vi "test.vi"(8 "error in (no error)":errorcluster, 11 "DAQOrcaFlash in":refnum<class "DAQOrcaFlash.lvclass">) -> (0 "error out":errorcluster, 3 "DAQOrcaFlash out":refnum<class "DAQOrcaFlash.lvclass">)   [LabVIEW 2012, in "DAQOrcaFlash.lvclass"]
uses:
  DAQOrcaFlash.lvclass
  <vilib>/vision/NI_Vision_Development_Module.lvlib
panel:
  out "max value 4":sgl
  out "min value 4":sgl
  out "max value 3":sgl
  out "min value 3":sgl
  out "min value":sgl
  out "max value":sgl
  in  "Path":path
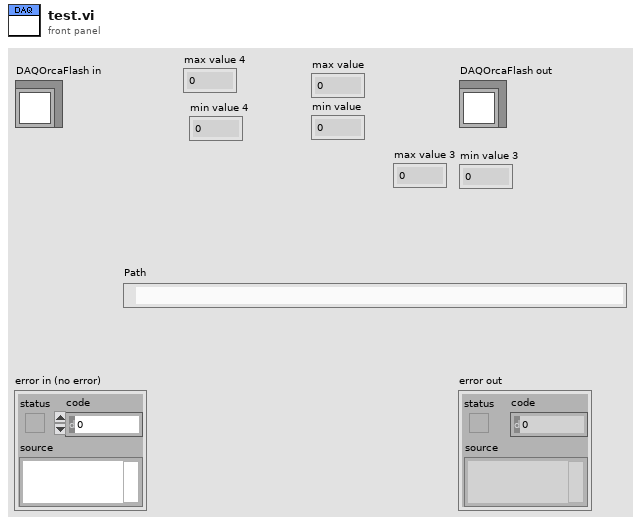
[diagram p1: front panel]
types:
  T1 = typedef "Image Type" = u32
  T2 = typedef "IMAQ Image.ctl" = refnum<image>
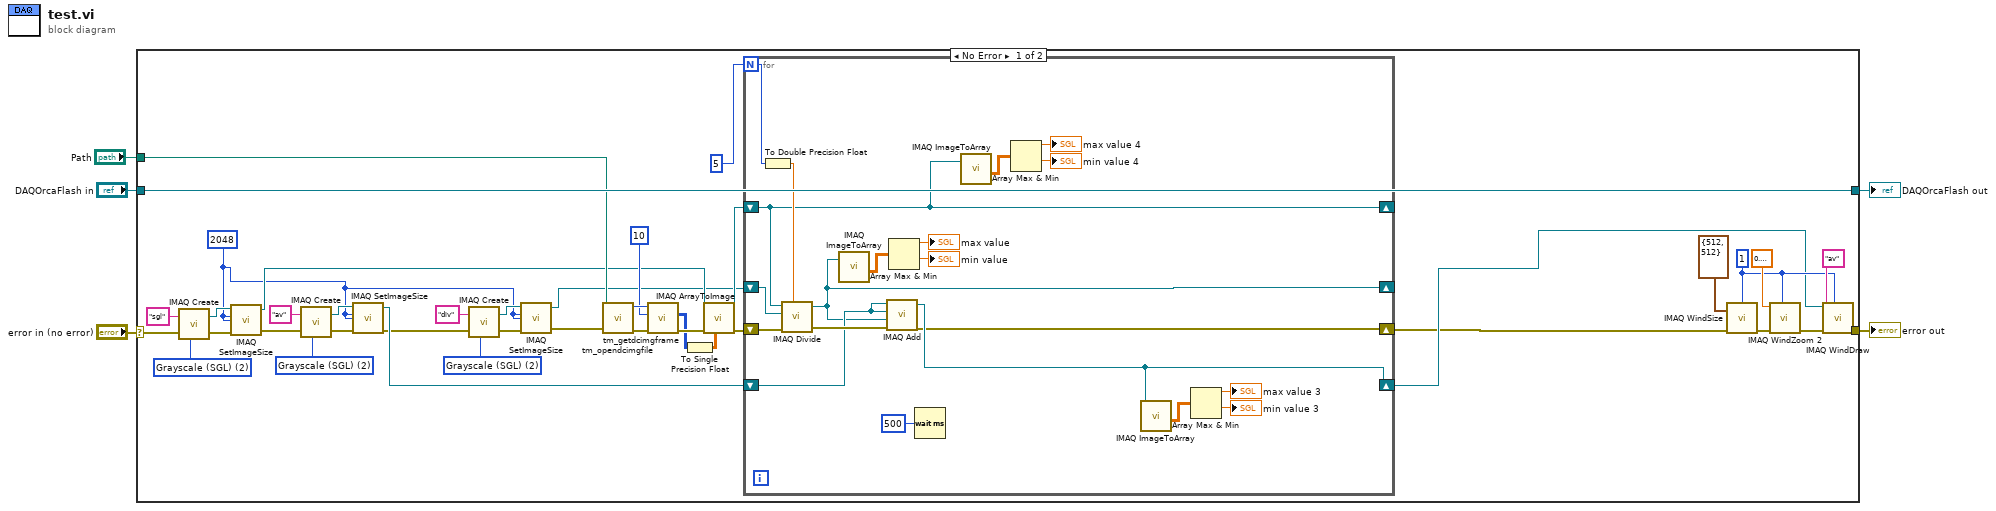
[diagram p0: block diagram]
diagram:
  n1 = case shown="No Error" "error in (no error)" {
    selector: "error in (no error)" -> [w37 w67]
    tunnel: [w24 w67] -> w4
    tunnel: [w45 w66] -> w2
    tunnel: "DAQOrcaFlash in" -> [w45 w66]
    tunnel: "Path" -> [w33 _]
    frame No Error {
      w13 = T1 2 items=["Grayscale (U8)", "Grayscale (I16)", "Grayscale (SGL)", "Complex (CSG)", "RGB (U32)", "HSL (U32)", "RGB (U64)", "Grayscale (U16)"] ("Image Type")
      w20 = T1 2 items=["Grayscale (U8)", "Grayscale (I16)", "Grayscale (SGL)", "Complex (CSG)", "RGB (U32)", "HSL (U32)", "RGB (U64)", "Grayscale (U16)"] ("Image Type")
      w8 = 2048 ("X Resolution")
      w40 = 1 ("Window Number")
      w43 = T1 2 items=["Grayscale (U8)", "Grayscale (I16)", "Grayscale (SGL)", "Complex (CSG)", "RGB (U32)", "HSL (U32)", "RGB (U64)", "Grayscale (U16)"] ("Image Type")
      n2 = call "IMAQ Create"("Image Name"="sgl", "Image Type"=w43, "error in (no error)"=w37) -> ("New Image"=w34:T2, "error out"=w35:errorcluster)  [unwired: 2 in]
      n3 = call "IMAQ SetImageSize"("error in (no error)"=w35, "Y Resolution"=w8, "X Resolution"=w8, "Image"=w34) -> ("error out"=w18:errorcluster, "Image Out"=w28:T2)  [unwired: 1 in]
      n4 = call "IMAQ Create"("Image Name"="av", "Image Type"=w20, "error in (no error)"=w18) -> ("New Image"=w22:T2, "error out"=w21:errorcluster)  [unwired: 2 in]
      n5 = call "IMAQ SetImageSize"("error in (no error)"=w21, "Y Resolution"=w8, "X Resolution"=w8, "Image"=w22) -> ("error out"=w10:errorcluster, "Image Out"=w17:T2)  [unwired: 1 in]
      n6 = call "IMAQ Create"("Image Name"="div", "Image Type"=w13, "error in (no error)"=w10) -> ("New Image"=w11:T2, "error out"=w12:errorcluster)  [unwired: 2 in]
      n7 = call "IMAQ SetImageSize"("error in (no error)"=w12, "Y Resolution"=w8, "X Resolution"=w8, "Image"=w11) -> ("error out"=w9:errorcluster, "Image Out"=w7:T2)  [unwired: 1 in]
      n8 = call <userlib>:"tm_opendcimgfile.vi"("error in (no error)"=w9, "Path"=w33) -> ("error out"=w30:errorcluster, "File Handle"=w32:u32)  [unwired: 7 in, 1 out]
      n9 = call <userlib>:"tm_getdcimgframe.vi"("error in (no error)"=w30, "Frame Index"=10, "File Handle in"=w32) -> ("error out"=w29:errorcluster, "Data"=w27:u16[][])  [unwired: 5 in, 2 out]
      n10 = To Single Precision Float(number=w27) -> (single precision float=w26:sgl[][])
      n11 = call "IMAQ ArrayToImage"("Image Pixels (Float)"=w26, "error in (no error)"=w29, "Image"=w28) -> ("error out"=w25:errorcluster, "Image Out"=w15:T2)  [unwired: 7 in]
      n12 = for {
        N: 5 -> [w53]
        shift-right: [w46] -> w6
        shift-left: w25 -> [w61]
        shift-right: [w55] -> w16
        shift-left: w17 -> [w52]
        shift-right: [w48] -> _
        shift-left: w15 -> [w48]
        shift-right: [w47] -> _
        shift-left: w7 -> [w54]
        n13 = To Double Precision Float(number=w53) -> (double precision float=w59:dbl)
        n14 = call "IMAQ Divide"("Image Src A"=w48, "Constant"=w59, "Image Dst"=w54, "error in (no error)"=w61) -> ("Image Dst Out"=w47:T2, "error out"=w60:errorcluster)  [unwired: 3 in]
        n15 = call "IMAQ ImageToArray"("Image"=w47) -> ("Image Pixels (Float)"=w64:sgl[][])  [unwired: 3 in, 4 out]
        n16 = call "IMAQ Add"("Image Src A"=w52, "Image Dst"=w52, "Image Src B"=w47, "error in (no error)"=w60) -> ("Image Dst Out"=w55:T2, "error out"=w46:errorcluster)  [unwired: 3 in]
        n17 = Array Max & Min(array=w64) -> (max value=→"max value":sgl, min value=→"min value":sgl)  [unwired: 2 out]
        n18 = Wait (ms)(milliseconds to wait=u32 500) -> ()  [unwired: 1 out]
        n19 = call "IMAQ ImageToArray"("Image"=w48) -> ("Image Pixels (Float)"=w51:sgl[][])  [unwired: 3 in, 4 out]
        n20 = Array Max & Min(array=w51) -> (max value=→"max value 4":sgl, min value=→"min value 4":sgl)  [unwired: 2 out]
        n21 = call "IMAQ ImageToArray"("Image"=w55) -> ("Image Pixels (Float)"=w56:sgl[][])  [unwired: 3 in, 4 out]
        n22 = Array Max & Min(array=w56) -> (max value=→"max value 3":sgl, min value=→"min value 3":sgl)  [unwired: 2 out]
      }
      n23 = call "IMAQ WindSize"("error in (no error)"=w6, "Width & Height"=cluster{"Width":i32, "Height":i32} {"Width"=512, "Height"=512}, "Window Number"=w40) -> ("error out"=w38:errorcluster)  [unwired: 3 in, 2 out]
      n24 = call "IMAQ WindZoom 2"("Window Number (0...15)"=w40, "error in (no error)"=w38, "Zoom Factor"=sgl 0.2) -> ("error out"=w39:errorcluster)  [unwired: 5 in, 3 out]
      n25 = call "IMAQ WindDraw"("Window Number (0...15)"=w40, "error in (no error)"=w39, "Title"="av", "Image"=w16) -> ("error out"=w24:errorcluster)  [unwired: 6 in, 1 out]
    }
    frame Error {
    }
  }
  "error out" <- w4
  "DAQOrcaFlash out" <- w2
